vi "Subsystem_Name_To_File_Path_Or_NT_Variable.vi"(2 "Enum String Name":string) -> (6 "Names":string, 7 "File Path":string, 8 "Values":string)   [LabVIEW 2019]
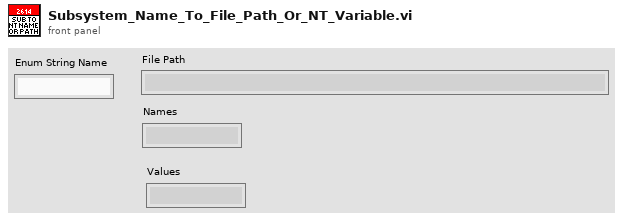
[diagram p1: front panel]
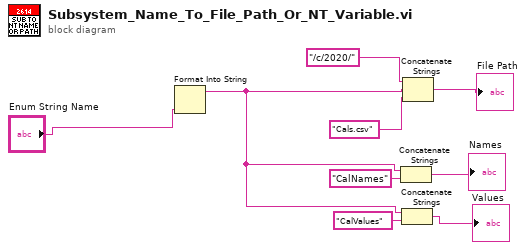
[diagram p0: block diagram]
diagram:
  n1 = Format Into String("Enum String Name") -> (resulting string=w4:string)  [unwired: 3 in, 1 out]
  n2 = Concatenate Strings(w4, "CalNames" ("string")) -> (→"Names":string)
  n3 = Concatenate Strings(w4, "CalValues" ("string")) -> (→"Values":string)
  n4 = Concatenate Strings("/c/2020/", w4, "Cals.csv") -> (→"File Path":string)
